vi "Get Previous Positions (config).vi"(8 "error in (no error)":errorcluster) -> (0 "error out":errorcluster, 3 "Previous Positions":dbl[](array[numeric]))   [LabVIEW 2020, in "ESP301.lvlib"]
uses:
  ESP301.lvlib
  <vilib>/Utility/config.llb/Read Key (String).vi
  <vilib>/Utility/config.llb/NI_LVConfig.lvlib
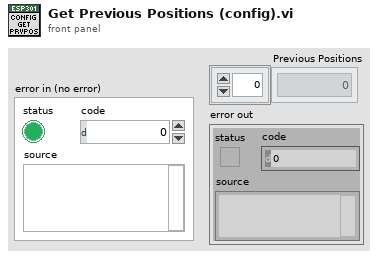
[diagram p1: front panel]
types:
  T1 = typedef "NI_LVConfig.lvlib/Config Data RefNum.ctl" = refnum<k1>
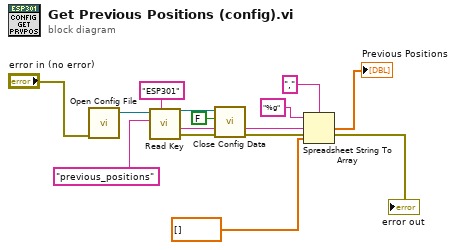
[diagram p0: block diagram]
diagram:
  n1 = call "Open Config File.vi"("error in (no error)"="error in (no error)") -> ("Refnum out"=w8:T1)  [unwired: 9 in, 1 out]
  n2 = call-poly <vilib>:"Read Key.vi"("section"="ESP301", "key"="previous_positions", "refnum"=w8) -> ("error out"=w11:errorcluster, "value"=w5:string, "refnum out"=w12:T1)  [unwired: 5 in, 1 out]
  n3 = call <vilib>:"Close Config Data.vi"("error in (no error)"=w11, "write file if changed (T)"=FALSE, "refnum"=w12) -> ("error out"=→"error out":errorcluster)  [unwired: 7 in, 1 out]
  n4 = Spreadsheet String To Array(delimiter (Tab)=",", format string="%g", spreadsheet string=w5, array type (2D Dbl)=dbl[] []) -> (array=→"Previous Positions":dbl[])
